vi "Create CDO Mode.vi"(7 "mode settings":T1, 8 "error in (no error)":errorcluster, 9 "number of channels":i32, 10 "channel settings":T2[](array[typedef]), 11 "counter driven output mode in":refnum<class "Counter Driven Output Mode.lvclass">) -> (0 "error out":errorcluster, 1 "channels":refnum<class "Counter Driven Output Channel.lvclass">[](array[class]), 3 "counter driven output mode out":refnum<class "Counter Driven Output Mode.lvclass">)   [LabVIEW 2017, in "Scan Engine Scripting.lvlib" / "Counter Driven Output Mode.lvclass"]
uses:
  Counter Driven Output Mode.lvclass
  Controls/counter driven output channel settings.ctl
  Channel Classes/Counter Driven Output Channel/Counter Driven State.ctl
  Drive from Slot.ctl
  Channel Classes/Counter Driven Output Channel/Counter Driven Output Channel.lvclass
  Scan Engine Scripting.lvlib
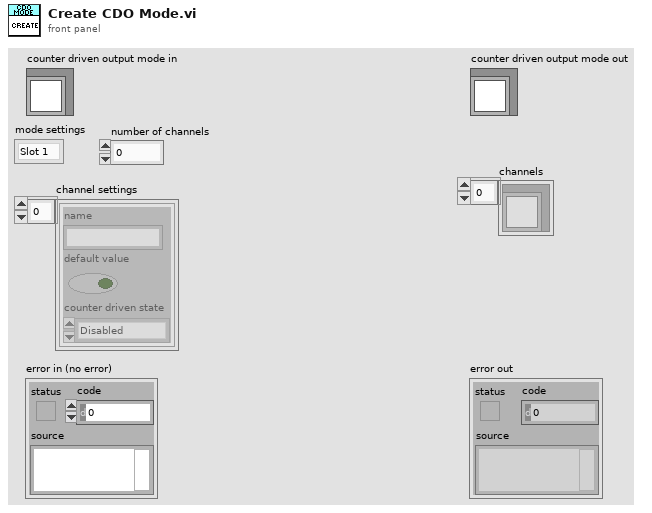
[diagram p1: front panel]
types:
  T1 = typedef "Scan Engine Scripting.lvlib/Counter Driven Output Mode.lvclass/Drive from Slot.ctl" = enum16{"Slot 1", "Slot 2", "Slot 3", "Slot 4", "Slot 5", "Slot 6", "Slot 7", "Slot 8"}
  T2 = typedef "Scan Engine Scripting.lvlib/counter driven output channel settings.ctl" = cluster{"name":string, "default value":bool, "counter driven state":T3}
  T3 = typedef "Scan Engine Scripting.lvlib/Counter Driven Output Channel.lvclass/Counter Driven State.ctl" = enum16{"Disabled", "Enabled"}
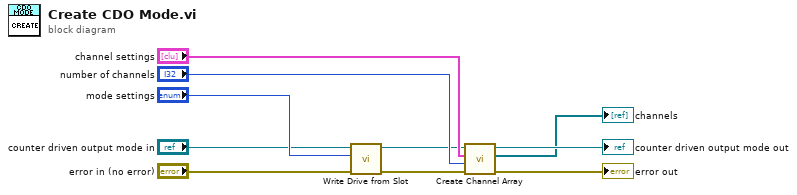
[diagram p0: block diagram]
diagram:
  n1 = call-dynamic "Write Drive from Slot.vi"("error in"="error in (no error)", "drive from slot"="mode settings", "counter driven output mode in"="counter driven output mode in") -> ("error out"=w1:errorcluster, "counter driven output mode out"=w6:refnum<class "Counter Driven Output Mode.lvclass">)  [unwired: 7 in]
  n2 = call "Create Channel Array.vi"("error in"=w1, "expected channel count"="number of channels", "channel settings"="channel settings", "counter driven output mode in"=w6) -> ("error out"=→"error out":errorcluster, "channels"=→"channels":refnum<class "Counter Driven Output Channel.lvclass">[], "counter driven output mode out"=→"counter driven output mode out":refnum<class "Counter Driven Output Mode.lvclass">)  [unwired: 5 in]
